vi "Registered user events.vi"() -> (1 "用户事件输出_Exit":refnum<user-event>, 2 "用户事件输出_侦听消息":refnum<user-event>, 3 "事件注册引用句柄":refnum<event-registration>)   [LabVIEW 2019, in "HTTP Server.lvlib"]
uses:
  HTTP Server.lvlib
  Listener Information.ctl
panel:
  in  "侦听消息":T1
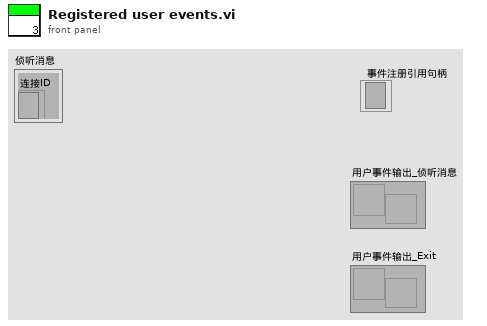
[diagram p1: front panel]
types:
  T1 = typedef "HTTP Server.lvlib/Listener Information.ctl" = cluster{"连接ID":refnum<k5>}
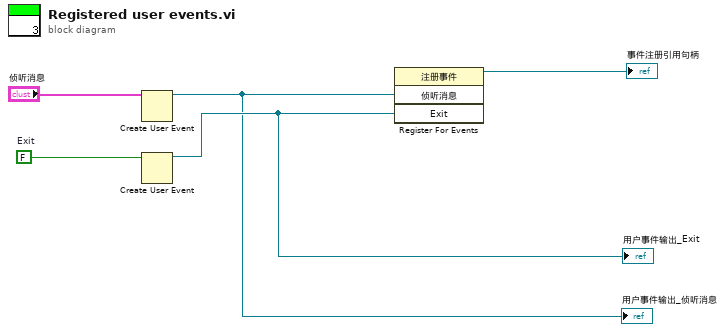
[diagram p0: block diagram]
diagram:
  w4 = FALSE  # Exit
  n1 = Create User Event(user event datatype="侦听消息") -> (user event=w1:refnum<user-event>)  [unwired: 1 in, 1 out]
  "用户事件输出_侦听消息" <- w1
  n2 = Create User Event ("创建用户事件")(user event datatype=w4) -> (user event=w3:refnum<user-event>)  [unwired: 1 in, 1 out]
  "用户事件输出_Exit" <- w3
  n3 = register-events(w1, w3) -> (reference out=→"事件注册引用句柄":refnum<event-registration>)  [unwired: 2 in, 1 out]
